vi "Read Waveform Measurement.vi"(8 "error in (no error)":errorcluster {"code" format="%.0x"}, 9 "Measurement Function (Rise Time)":string(combo)="RISETIME", 10 "Channel (\"Channel 1\")":string(combo)="CHAN1", 11 "VISA Resource Name":refnum<visa-resource-name>) -> (0 "error out":errorcluster {"code" format="%.0x"}, 2 "measurement":dbl caption="Measurement" format="%^.2e", 3 "VISA Resource Name Out":refnum<visa-resource-name>)   [LabVIEW 2011, in "Agilent 546XX Series.lvlib"]
doc: "This VI obtains a waveform measurement and returns the measurement value. You specify a particular measurement type, such as rise time, frequency, and voltage peak-to-peak. The waveform on which the oscilloscope calculates the waveform measurement is from an acquisition that you previously initiated. \n\nUse the ag546xx Initiate Acquisition VI, ag546xx Read Waveform VI, or ag546xx Read Min Max Waveform VI to start an acquisition on the channels that you enable with the ag546xx Configure Channel VI. You call this VI separately for each waveform measurement you want to obtain on a specific channel."
uses:
  Agilent 546XX Series.lvlib
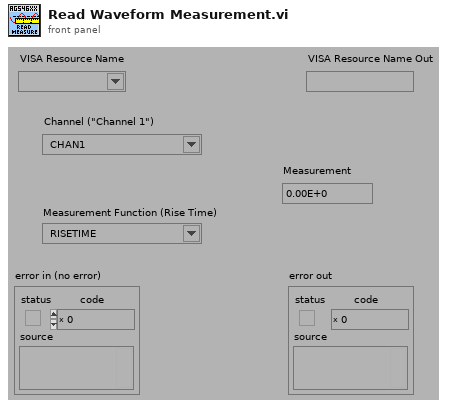
[diagram p1: front panel]
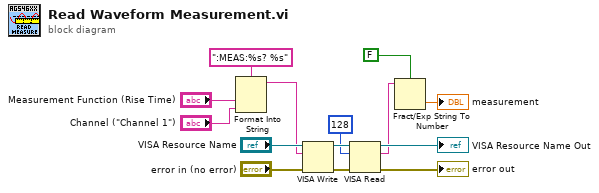
[diagram p0: block diagram]
diagram:
  n1 = Format Into String(format string=":MEAS:%s? %s", "Measurement Function (Rise Time)", "Channel (\"Channel 1\")") -> (resulting string=w5:string)  [unwired: 2 in, 1 out]
  n2 = VISA Write(VISA resource name="VISA Resource Name", write buffer=w5, error in (no error)="error in (no error)") -> (VISA resource name out=w14:refnum<visa-resource-name>, error out=w13:errorcluster)  [unwired: 1 out]
  n3 = VISA Read(VISA resource name=w14, byte count=u32 128, error in (no error)=w13) -> (VISA resource name out=→"VISA Resource Name Out":refnum<visa-resource-name>, read buffer=w3:string, error out=→"error out":errorcluster)  [unwired: 1 out]
  n4 = Fract/Exp String To Number(use system decimal point (T)=FALSE, string=w3) -> (number=→"measurement":dbl)  [unwired: 2 in, 1 out]
